vi "TOML example write section.vi"() -> ()   [LabVIEW 2017]
doc: "This example demonstrates how to parse a TOML file"
uses:
  d02ca0be-f060-482f-a67e-ed4f3b17e19f.vi
  <userlib>/LV-TOML/lib/TOML to LabVIEW.vi
  lib/TOML.lvlib
panel:
  out "LV to TOML error":errorcluster
  in  "Error if missing element":bool
  out "TOML to LV error":errorcluster
  in  "Parsed Data":T1
  out "new TOML String":string
  in  "original TOML String":string
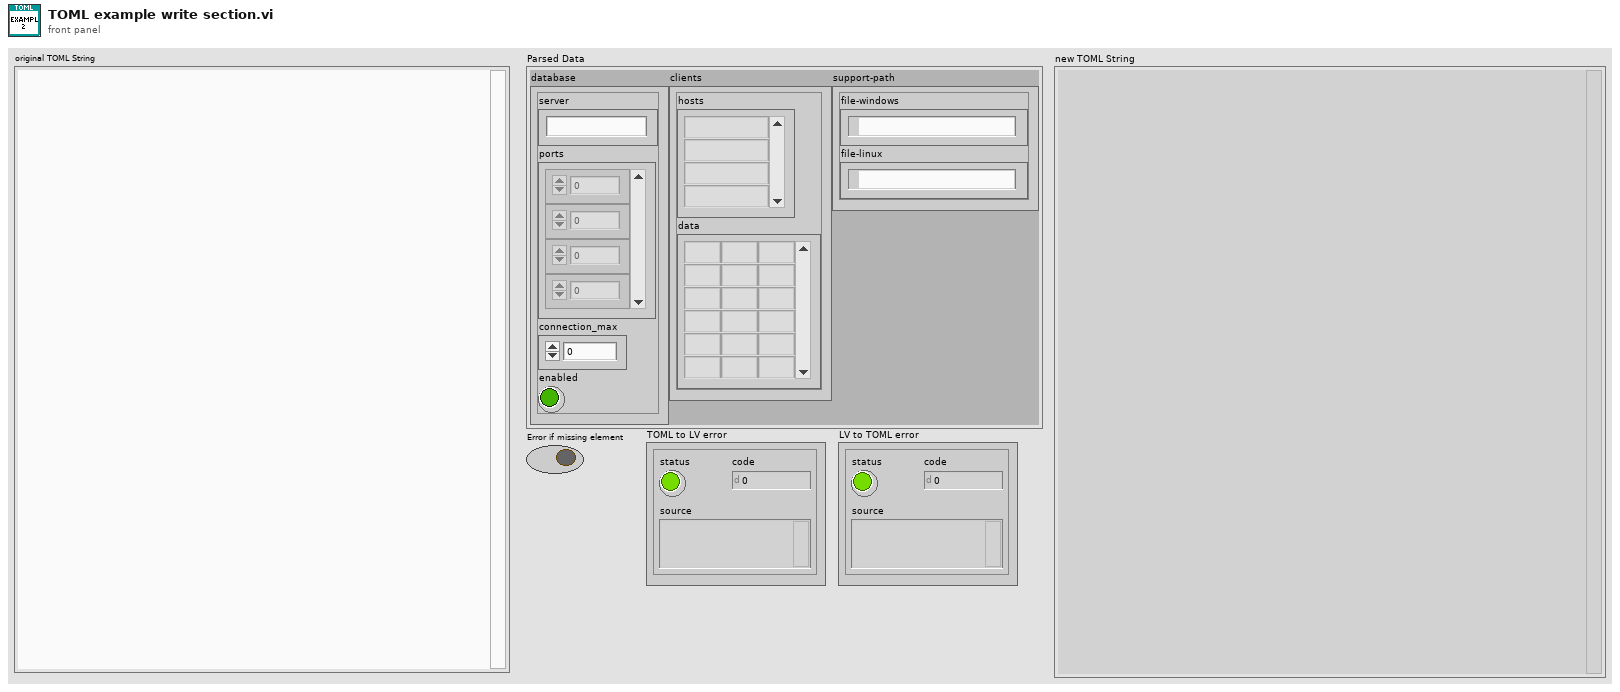
[diagram p1: front panel]
types:
  T1 = cluster{"database":cluster{"server":string, "ports":u16[], "connection_max":dbl, "enabled":bool}, "clients":cluster{"hosts":string[], "data":string[][]}, "support-path":cluster{"file-windows":path, "file-linux":path}}
  T2 = typedef "TOML.lvlib/TOML Value.ctl" = cluster{"type":enum16{"Table", "Array", "String", "Integer", "Float", "Boolean", "Offset Date-Time", "Local Date-Time", "Local Date", "Local Time", "Path"}, "value":variant}
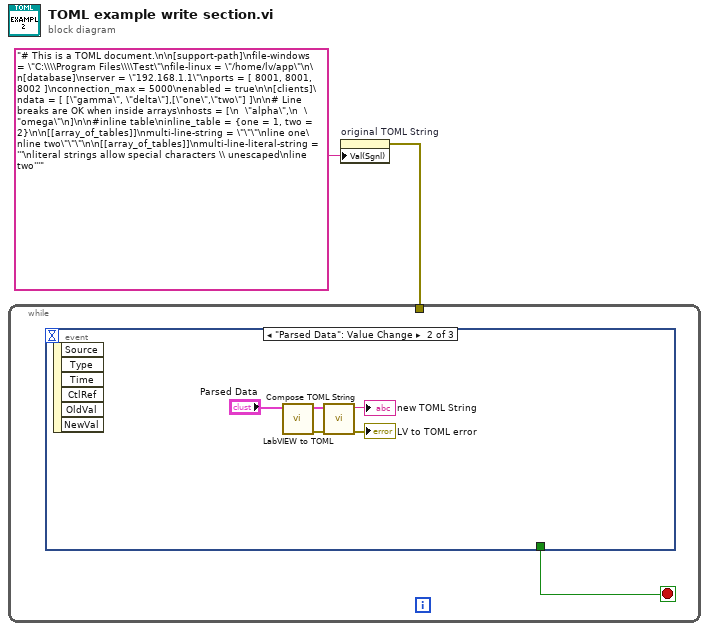
[diagram p0: block diagram]
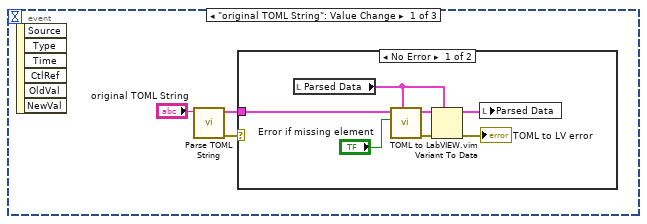
[diagram p2: hidden frame]
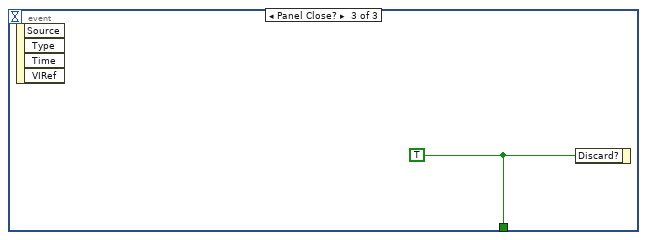
[diagram p4: hidden frame]
diagram:
  n1 = property on="original TOML String" class="Str"("Val(Sgnl)"="# This is a TOML document.\n\n[support-path]\nfile-windows = \"C:\\\\Program Files\\\\Test\"\nfile-linux = \"/home/lv/app\"\n\n[database]\nserver = \"192.168.1.1\"\nports = [ 8001, 8001, 8002 ]\nconnection_max = 5000\nenabled = true\n\n[clients]\ndata = [ [\"gamma\", \"delta\"],[\"one\",\"two\"] ]\n\n# Line breaks are OK when inside arrays\nhosts = [\n  \"alpha\",\n  \"omega\"\n]\n\n#inline table\ninline_table = {one = 1, two = 2}\n\n[[array_of_tables]]\nmulti-line-string = \"\"\"\nline one\nline two\"\"\"\n\n[[array_of_tables]]\nmulti-line-literal-string = '''\nliteral strings allow special characters \\ unescaped\nline two'''" ("TOML String")) -> (error out=w1:errorcluster)  [unwired: 2 in, 1 out]
  n2 = while {
    tunnel: w1 -> [_]
    stop <- w3 stop-if-true
    n3 = event shown="[1] \"Parsed Data\": Value Change" {
      selector: _ -> [_ _ _]
      dyn-events: _ -> [_ _ _]
      timeout: _ -> [_ _ _]
      tunnel: [_ _ w19] -> w3
      event "original TOML String": Value Change {
        n4 = event-data() -> ()  [unwired: 1 in, 6 out]
        n5 = call "Parse TOML String.vi"("String"="original TOML String") -> ("error out"=w6:errorcluster, "Value"=w4:T2)  [unwired: 9 in]
        n6 = case shown="No Error" w6 {
          tunnel: w4 -> [w12 _]
          frame No Error {
            n7 = local read "Parsed Data"() -> (w13:T1)
            n8 = call "TOML to LabVIEW.vim"("datatype"=w13, "Error if missing element"="Error if missing element", "Value"=w12) -> ("error out"=w10:errorcluster, "LV Data"=w11:T1)  [unwired: 6 in, 1 out]
            n9 = Variant To Data(error in=w10, type=w13, Variant=w11) -> (data=w8:T1, error out=→"TOML to LV error":errorcluster)
            n10 = local write "Parsed Data"(w8) -> ()
          }
          frame Error {
          }
        }
      }
      event "Parsed Data": Value Change {
        n11 = event-data() -> ()  [unwired: 1 in, 6 out]
        n12 = call "LabVIEW to TOML.vi"("LV Value"="Parsed Data") -> ("error out"=w15:errorcluster, "TOML Value"=w16:T2)  [unwired: 9 in]
        n13 = call "Compose TOML String.vi"("error in (no error)"=w15, "Value"=w16) -> ("error out"=→"LV to TOML error":errorcluster, "String"=→"new TOML String":string)  [unwired: 8 in]
      }
      event Panel Close? {
        w19 = TRUE
        n14 = event-data() -> ()  [unwired: 1 in, 4 out]
        n15 = event-data("Discard?"=w19) -> ()  [unwired: 1 in, 1 out]
      }
    }
  }
